vi "dfd_SOS_Direct_IIR_II_T_C.vi"() -> ()   [LabVIEW 2017, in "NI_DigFilterTemp.lvlib"]
uses:
  <vilib>/addons/Digital Filter Design/NI_DigFilterTemp.lvlib
panel:
  in  "String":string="\n\n/* ---- Constants ----*/\n#define %CapName%_N_SECTIONS %kSection%\n#define %CapName%_N_STATES (2*%CapName%_N_SECTIONS)\n#define %CapName%_N_COEFA (2*%CapName%_N_SECTIONS)\n#define %CapName%_N_COEFB (3*%CapName%_N_SECTIONS)\n\n/* ---- Global Variables Declaration ----*/\nstatic %CoefAType% %FilterBlkName%_CoefA[%CapName%_N_COEFA];\nstatic %CoefBType% %FilterBlkName%_CoefB[%CapName%_N_COEFB];\n%InternalFunctionsDeclaration%\n\n%ShiftDefine%\n\n%AssistantFunctions%\n\n/* ---- Implement the Fixed-Point Filter ---- */\n%OutType% %FilterBlkName%_Filtering (%InType% sampleIn, %FilterBlkName%_State state)\n{\n\tI32 accA, accB;\n\t%MultType% mult_a, mult_b;\n\tint i;    \n\tint iA, iB;\n\n\taccA = (%I32TypeCast%sampleIn << IN2SUM);\n\n\tiA = iB = 0;\n\tfor (i=0; i < %CapName%_N_SECTIONS; i++)\n\t{\n\t\tmult_b = %PreMultCast%(accA << SUM2MULT);\n\n\t\t/* Filtering */\n\t\taccA = (%FilterBlkName%_%MultB%(mult_b, %FilterBlkName%_CoefB[iB++]) << PROD2SUM);\n\t\taccA += (state[iA] << DELAY2SUM);\n\n\t\tmult_a = %PreMultCast%(accA << SUM2MULT);\n\n\t\t/* Update the internal states */\n\t\taccB = (state[iA+1] << DELAY2SUM);\n\t\taccB += (%FilterBlkName%_%MultB%(mult_b, %FilterBlkName%_CoefB[iB++]) << PROD2SUM);\n\t\taccB -= (%FilterBlkName%_%MultA%(mult_a, %FilterBlkName%_CoefA[iA]) << PROD2SUM);\n\t\tstate[iA++] = (accB << SUM2DELAY);\n\n\t\taccB = (%FilterBlkName%_%MultB%(mult_b, %FilterBlkName%_CoefB[iB++]) << PROD2SUM);\n\t\taccB -= (%FilterBlkName%_%MultA%(mult_a, %FilterBlkName%_CoefA[iA]) << PROD2SUM);\n\t\tstate[iA++] = (accB << SUM2DELAY);\n\t}\n\n\t%ApplyGainAccA%\n\n\treturn (%OutType%)accA;\n}\n\n/* ---- Internal Functions ---- */\n%InternalFunctions%\n\n/* ---- Filter Coefficients ---- */\nstatic %CoefAType% %FilterBlkName%_CoefA [] = {\n%CoefficientsA%\n};\nstatic %CoefBType% %FilterBlkName%_CoefB [] = {\n%CoefficientsB%\n};\n"
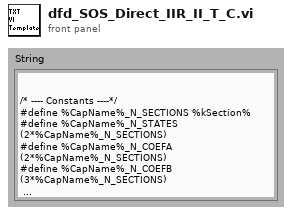
[diagram p1: front panel]
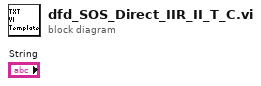
[diagram p0: block diagram]
diagram:
